vi "Brushed DC Motor.vi"() -> ()   [LabVIEW 2019]
doc: "The NI ELVIS III Custom FPGA Project template acquires button data from the onboard button and displays the button value on a Boolean indicator."
uses:
  <vilib>/Platform/TimedLoop/XDataNode/timing_clust.ctl
  <vilib>/Platform/TimedLoop/XDataNode/nitl_modes.ctl
  <vilib>/Platform/TimedLoop/XDataNode/wakeup.ctl
  <vilib>/Platform/TimedLoop/XDataNode/XDataNode.xnode
  <vilib>/Platform/TimedLoop/XDataNode/XDNodeRunTimeDep.lvlib
panel:
  out "Error Out":errorcluster
  out "Brushed DC Motor \nSpeed (RPM)":dbl format="%#.0f"
  out "Brushed DC Motor Speed":dbl(graph)
  in  "Brushed DC Motor Voltage":sgl(knob) min=-5 max=5 step=0.01 scale=-5.0..5.0
  in  "Stop Button":bool
  # "Mechatronic Actuators Board"
  # "Brushed DC Motor"
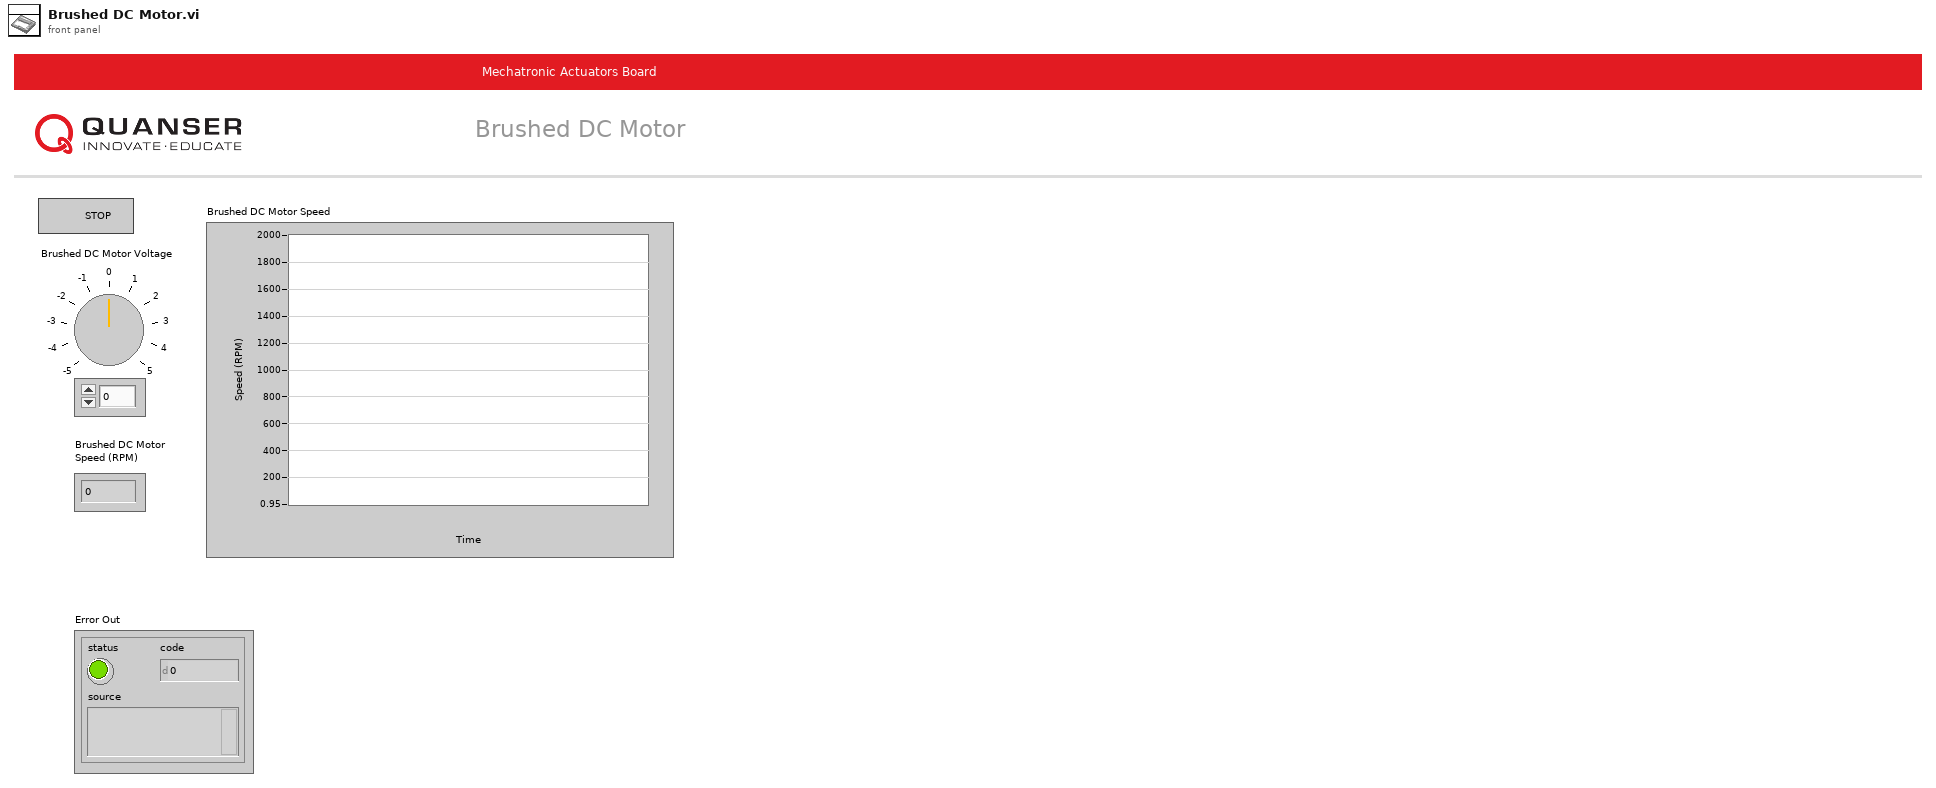
[diagram p1: front panel]
types:
  T1 = typedef "XDNodeRunTimeDep.lvlib/timing_clust.ctl" = cluster{"Expected End [f-1]":u64, "Actual End [f-1]":u64, "Finished Late? [f-1]":bool, "Expected End [i-1]":u64, "Actual End [i-1]":u64, "Finished Late? [i-1]":bool, "Expected Start [i]":u64, "Actual Start [i]":u64, "Expected Start [f]":u64, "Actual Start [f]":u64, "Source Name":string, "Structure Name":string, "Period":i64, "Deadline":i64, "Offset":i64, "Start":i64, "Priority":i32, "Timeout":i32, "Mode":T2, "Wakeup Reason":T3, "Error":errorcluster, "Source Type":string, "Secondary Source Type":string, "Global End Time":u64, "Global Start Time":u64, "Frame Duration":u64, "Iteration Duration":u64, "Assigned CPU":i32, "I/O Scan Engine Mode":u32}
  T2 = typedef "XDNodeRunTimeDep.lvlib/nitl_modes.ctl" = enum32{"No Change", "Process missed periods, maintain original phase", "Discard missed periods, maintain original phase", "Process missed periods, ignore original phase", "Discard missed periods, ignore original phase"}
  T3 = typedef "XDNodeRunTimeDep.lvlib/wakeup.ctl" = enum32{"Normal", "Aborted", "Asynchronous wakeup", "Timing source error", "Timed loop error", "Timeout"}
  T4 = typedef "Actuators IO Cluster.ctl" = cluster{"Error":errorcluster, "FPGA Ref":refnum<k20>}
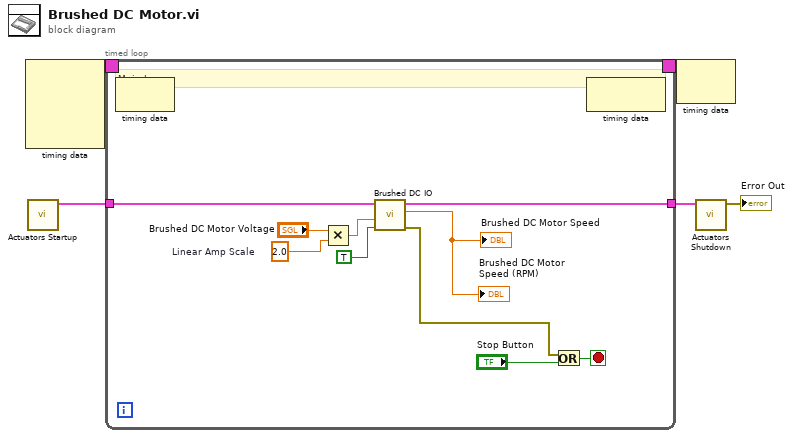
[diagram p0: block diagram]
diagram:
  n1 = node-c288() -> (w5:T1)  [unwired: 4 in]
  n2 = call "Actuators Startup.vi"() -> ("IO Cluster OUT"=w3:T4)  [unwired: 11 in]
  n3 = timed-loop {
    timing: w5 -> [_]
    timing-out: [_] -> w4
    tunnel: w3 -> [w13]
    tunnel: [w12] -> w2
    stop <- w15 stop-if-true
    w8 = sgl 2.0  # Linear Amp Scale
    # "Main Loop"
    n4 = node-c288() -> ()  [unwired: 1 in, 1 out]
    n5 = Multiply(x="Brushed DC Motor Voltage", y=w8) -> (x*y=w7:sgl)
    n6 = call "Brushed DC IO.vi"("Linear Amplifier Enable"=TRUE, "Brushed DC Motor Linear"=w7, "IO Cluster IN"=w13) -> ("Error Out"=w11:errorcluster, "Brushed DC Motor Speed (RPM)"=→"Brushed DC Motor Speed" →"Brushed DC Motor \nSpeed (RPM)":dbl, "IO Cluster OUT"=w12:T4)  [unwired: 5 in, 1 out]
    n7 = Or(x=w11, y="Stop Button") -> (x .or. y?=w15:bool)
    n8 = node-c288() -> ()  [unwired: 1 in, 1 out]
  }
  n9 = node-c288(w4) -> ()  [unwired: 1 out]
  n10 = call "Actuators Shutdown.vi"("IO Cluster IN"=w2) -> ("Error Out"=→"Error Out":errorcluster)  [unwired: 10 in]
